vi "_Update Mass Range.vi"(4 "error in":errorcluster, 5 "Mass Range":T1 {"Resolution Type" items=["High/High", "Medium/Medium", "Low/Low", "High/Medium", "High/Low", "Medium/High", "Medium/Low", "Low/High", "Low/Medium"]}, 6 "Offset":u16) -> (0 "error out":errorcluster, 2 "Next Offset":u16)   [LabVIEW 2015]
uses:
  Type/_RT Mass Range.ctl
  Type/_RT Res Type.ctl
  Type/_RT Active Ch.ctl
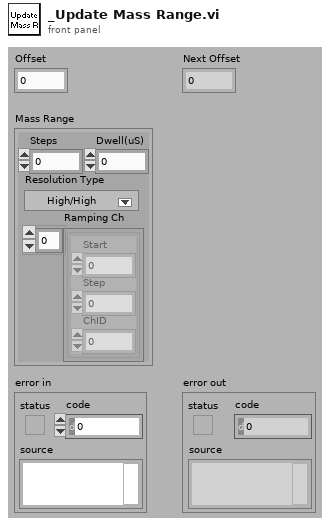
[diagram p1: front panel]
types:
  T1 = typedef "_RT Mass Range.ctl" = cluster{"Steps":i32, "Dwell(uS)":i32, "Resolution Type":T2, "Ramping Ch":T3[]}
  T2 = typedef "_RT Res Type.ctl" = u16
  T3 = typedef "_RT Active Ch.ctl" = cluster{"Start":i32, "Step":i32, "ChID":i32}
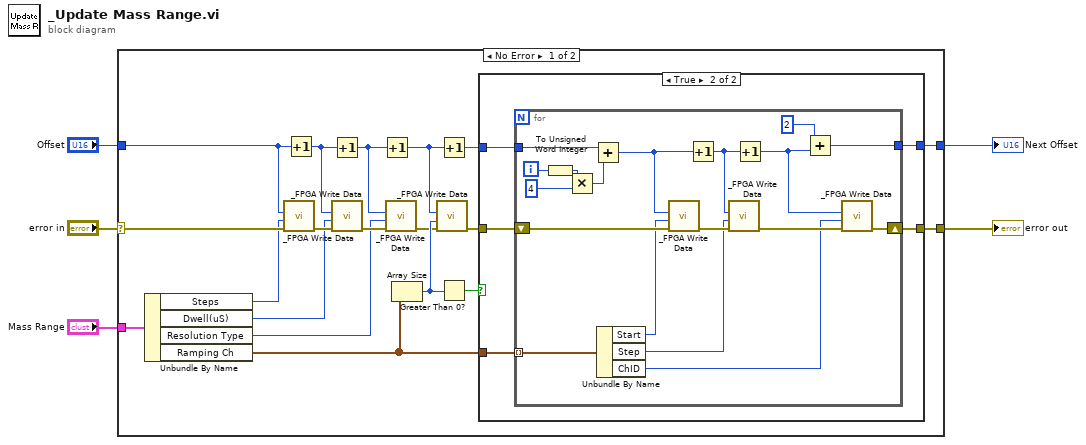
[diagram p0: block diagram]
diagram:
  n1 = case shown="No Error" "error in" {
    selector: "error in" -> [w23 w51]
    tunnel: [w15 w51] -> w4
    tunnel: "Offset" -> [w19 w50]
    tunnel: [w13 w50] -> w2
    tunnel: "Mass Range" -> [w6 _]
    frame No Error {
      n2 = Unbundle By Name(w6) -> ("Steps"=w22:i32, "Dwell(uS)"=w20:i32, "Resolution Type"=w9:T2, "Ramping Ch"=w12:T3[])
      n3 = call "_FPGA Write Data.vi"("error in"=w23, "Data"=w22, "Address"=w19) -> ("error out"=w24:errorcluster)  [unwired: 3 in, 2 out]
      n4 = Increment(x=w19) -> (x+1=w21:u16)
      n5 = Increment(x=w21) -> (x+1=w10:u16)
      n6 = call "_FPGA Write Data.vi"("error in"=w24, "Data"=w20, "Address"=w21) -> ("error out"=w11:errorcluster)  [unwired: 3 in, 2 out]
      n7 = Increment(x=w10) -> (x+1=w7:u16)
      n8 = call "_FPGA Write Data.vi"("error in"=w11, "Data"=w9, "Address"=w10) -> ("error out"=w8:errorcluster)  [unwired: 3 in, 2 out]
      n9 = Array Size(array=w12) -> (size(s)=w18:i32)
      n10 = call "_FPGA Write Data.vi"("error in"=w8, "Data"=w18, "Address"=w7) -> ("error out"=w16:errorcluster)  [unwired: 3 in, 2 out]
      n11 = Increment(x=w7) -> (x+1=w14:u16)
      n12 = Greater Than 0?(x=w18) -> (x > 0?=w17:bool)
      n13 = case shown="True" w17 {
        tunnel: [w26 w28] -> w15
        tunnel: w16 -> [w26 w30]
        tunnel: w14 -> [w25 w29]
        tunnel: [w25 w27] -> w13
        tunnel: w12 -> [_ w31]
        frame False {
        }
        frame True {
          n14 = for {
            tunnel: w31 -> [w45] mode=indexing
            shift-right: [w36] -> w28
            shift-left: w30 -> [w44]
            tunnel: w29 -> [w46]
            tunnel: [w34] -> w27
            i -> [w49]
            n15 = To Unsigned Word Integer(number=w49) -> (unsigned 16bit integer=w32:u16)
            n16 = Multiply(x=w32, y=u16 4) -> (x*y=w47:u16)
            n17 = Add(x=w46, y=w47) -> (x+y=w40:u16)
            n18 = Unbundle By Name(w45) -> ("Start"=w43:i32, "Step"=w41:i32, "ChID"=w37:i32)
            n19 = call "_FPGA Write Data.vi"("error in"=w44, "Data"=w43, "Address"=w40) -> ("error out"=w42:errorcluster)  [unwired: 3 in, 2 out]
            n20 = Increment(x=w40) -> (x+1=w38:u16)
            n21 = call "_FPGA Write Data.vi"("error in"=w42, "Data"=w41, "Address"=w38) -> ("error out"=w39:errorcluster)  [unwired: 3 in, 2 out]
            n22 = Increment(x=w38) -> (x+1=w35:u16)
            n23 = Add(x=u16 2, y=w35) -> (x+y=w34:u16)
            n24 = call "_FPGA Write Data.vi"("error in"=w39, "Data"=w37, "Address"=w35) -> ("error out"=w36:errorcluster)  [unwired: 3 in, 2 out]
          }
        }
      }
    }
    frame Error {
    }
  }
  "error out" <- w4
  "Next Offset" <- w2
